vi "Change Case Structure to Error case structure.vi"(6 "Variant in":variant, 7 "Shift Pressed?":bool, 8 "error in (no error)":errorcluster, 10 "QD Combo Box Ref":refnum<vi>, 11 "QD Launch VI Ref":refnum<vi>) -> (0 "error out":errorcluster, 4 "Variant out":variant)   [LabVIEW 2014]
doc: "Write a 1-2 sentence description of the functionality of your plugin here. Replace the \"$\" below with the character you wish to assign as the default shortcut for this plugin. Do not add any text after the 'Default Shortcut' line below.\n\nDefault Shortcut - [E]"
panel:
  in  "Undo Name":string="Quick Drop Keyboard Shortcut"
  # "Do not change the connector pane of this VI.\n\nSee the block diagram for directions on how to use this template."
  # "Specify the name of the Undo transaction"
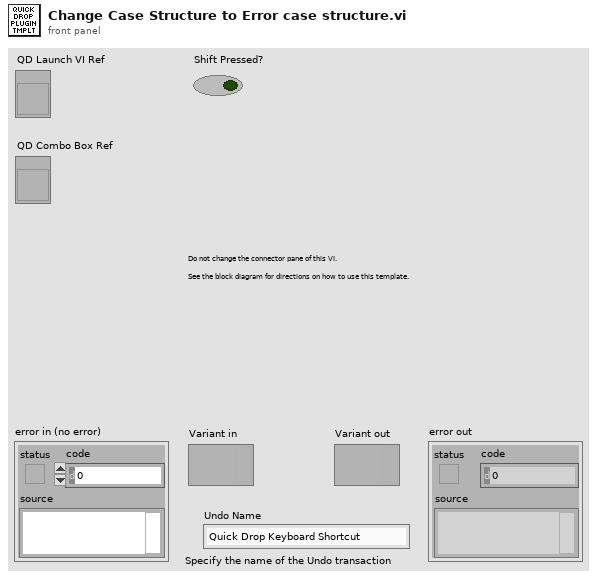
[diagram p1: front panel]
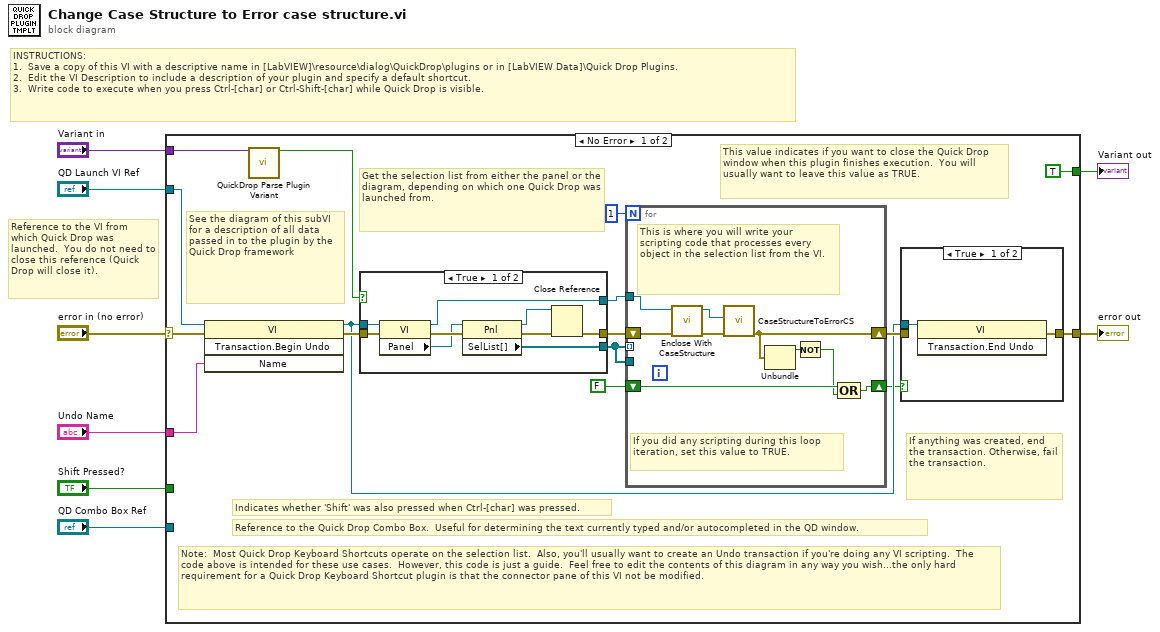
[diagram p0: block diagram]
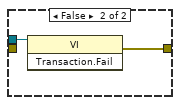
[diagram p2: hidden frame]
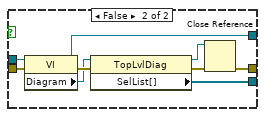
[diagram p3: hidden frame]
diagram:
  # "Reference to the VI from which Quick Drop was launched.  You do not need to close this reference (Quick Drop will close it)."
  # "INSTRUCTIONS:\n1.  Save a copy of this VI with a descriptive name in [LabVIEW]\\resource\\dialog\\QuickDrop\\plugins or in [LabVIEW Data]\\Quick Drop Plugins.\n2.  Edit the VI Description to include a description of your plugin and specify a default shortcut. \n3.  Write code to execute when you press Ctrl-[char] or Ctrl-Shift-[char] while Quick Drop is visible."
  n1 = case shown="No Error" "error in (no error)" {
    selector: "error in (no error)" -> [w23 w56]
    tunnel: [w17 w56] -> w7
    tunnel: "QD Launch VI Ref" -> [w22 _]
    tunnel: "Shift Pressed?" -> [_ _]
    tunnel: "QD Combo Box Ref" -> [_ _]
    tunnel: "Variant in" -> [w24 _]
    tunnel: "Undo Name" -> [w21 _]
    tunnel: [TRUE _] -> w1
    frame No Error {
      # "Note:  Most Quick Drop Keyboard Shortcuts operate on the selection list.  Also, you'll usually want to create an Undo transaction if you're doing any VI scripting.  The code above is intended for these use cases.  However, this code is just a guide.  Feel free to edit the contents of this diagram in any way you wish...the only hard requirement for a Quick Drop Keyboard Shortcut plugin is that the connector pane of this VI not be modified."
      # "Get the selection list from either the panel or the diagram, depending on which one Quick Drop was launched from."
      # "If anything was created, end the transaction. Otherwise, fail the transaction."
      # "This value indicates if you want to close the Quick Drop window when this plugin finishes execution.  You will usually want to leave this value as TRUE."
      # "See the diagram of this subVI for a description of all data passed in to the plugin by the Quick Drop framework"
      # "Reference to the Quick Drop Combo Box.  Useful for determining the text currently typed and/or autocompleted in the QD window."
      # "Indicates whether 'Shift' was also pressed when Ctrl-[char] was pressed."
      n2 = invoke class="VI" method="Transaction.Begin Undo"(reference=w22, error in=w23, "Name"=w21) -> (reference out=w14:refnum<vi>, error out=w18:errorcluster)  [unwired: 1 in, 2 out]
      n3 = call <vilib>:"QuickDrop Parse Plugin Variant.vi"("QDKS Variant in"=w24) -> ("QD Launch VI Panel?"=w19:bool)  [unwired: 12 in, 2 out]
      n4 = case shown="True" w19 {
        tunnel: w18 -> [w46 w55]
        tunnel: w14 -> [w45 w54]
        tunnel: [w40 w49] -> w16
        tunnel: [w39 w48] -> w10
        tunnel: [w38 w47] -> w9
        frame True {
          n5 = property class="VI"(reference=w45, error in=w46) -> (reference out=w38:refnum<vi>, error out=w44:errorcluster, "Panel"=w43:refnum<vi>)
          n6 = property class="Pnl"(reference=w43, error in=w44) -> (reference out=w41:refnum<vi>, error out=w42:errorcluster, "SelList[]"=w39:refnum<vi>[])
          n7 = Close Reference(reference=w41, error in (no error)=w42) -> (error out=w40:errorcluster)
        }
        frame False {
          n8 = property class="VI"(reference=w54, error in=w55) -> (reference out=w47:refnum<vi>, error out=w53:errorcluster, "Diagram"=w52:refnum<vi>)
          n9 = property class="TopLvlDiag"(reference=w52, error in=w53) -> (reference out=w50:refnum<vi>, error out=w51:errorcluster, "SelList[]"=w48:refnum<vi>[])
          n10 = Close Reference(reference=w50, error in (no error)=w51) -> (error out=w49:errorcluster)
        }
      }
      n11 = for {
        N: 1 -> [_]
        shift-right: [w27] -> w15
        shift-left: w16 -> [w31]
        shift-right: [w32] -> w12
        shift-left: FALSE -> [w33]
        tunnel: w10 -> [_] mode=indexing
        tunnel: w10 -> [_]
        tunnel: w9 -> [w28]
        # "This is where you will write your scripting code that processes every object in the selection list from the VI."
        # "If you did any scripting during this loop iteration, set this value to TRUE."
        n12 = call <resource>:"Enclose With CaseStructure.vi"("error in (no error)"=w31, "QD Launch VI Ref"=w28) -> ("error out"=w30:errorcluster, "EncloseSelection2"=w29:refnum<vi>)  [unwired: 8 in]
        n13 = call <resource>:"CaseStructureToErrorCS.vi"("error in (no error)"=w30, "reference"=w29) -> ("error out"=w27:errorcluster)  [unwired: 9 in]
        n14 = Unbundle(w27) -> ("status"=w26:bool)  [unwired: 2 out]
        n15 = Not(x=w26) -> (.not. x?=w25:bool)
        n16 = Compound Arithmetic op=OR(w33, w25) -> (w32:bool)
      }
      n17 = case shown="True" w12 {
        tunnel: w14 -> [w34 w36]
        tunnel: [w35 w37] -> w17
        tunnel: w15 -> [_ _]
        frame True {
          n18 = invoke class="VI" method="Transaction.End Undo"(reference=w34) -> (error out=w35:errorcluster)  [unwired: 2 in, 2 out]
        }
        frame False {
          n19 = invoke class="VI" method="Transaction.Fail"(reference=w36) -> (error out=w37:errorcluster)  [unwired: 2 in, 2 out]
        }
      }
    }
    frame Error {
    }
  }
  "error out" <- w7
  "Variant out" <- w1
